vi "Set Bias Voltage.vi"(8 "error in (no error)":errorcluster, 9 "Channel":i32, 10 "Bias Voltage (V)":dbl, 11 "Example in":refnum<class "Instrument.Template.lvclass">) -> (0 "error out":errorcluster, 3 "Example out":refnum<class "Instrument.Template.lvclass">)   [LabVIEW 2019, in "Instrument.Template.lvclass"]
uses:
  Instrument.Template/Instrument.Template.lvclass
  Typedefs/Instrument.Template.Commands--Enum.ctl
  67792bfe-8e2c-4879-abc2-cb448bcec168.vi
  67792bfe-8e2c-4879-abc2-cb448bcec168.vi/c75e12d4-2661-49a5-9afc-dbffdb694870.vi
  67792bfe-8e2c-4879-abc2-cb448bcec168.vi/2a0bf3c4-890a-488b-bba9-7d0e50155bd9.vi
  67792bfe-8e2c-4879-abc2-cb448bcec168.vi/2a0bf3c4-890a-488b-bba9-7d0e50155bd9.vi/a640b9e0-2bb1-42d0-9491-26b19c1d8e7b.vi
  67792bfe-8e2c-4879-abc2-cb448bcec168.vi/2a0bf3c4-890a-488b-bba9-7d0e50155bd9.vi/8610e4ee-7e05-4c89-86eb-49a2000bc7ea.vi
  SMOs/RemoteControl/API/Remote Client.vi
  <vilib>/JDP Science/JSONtext/JSON text to Variant.vi
  <vilib>/JDP Science/JSONtext/LVClass Serializer/JSONtext LVClass Serializer.lvclass
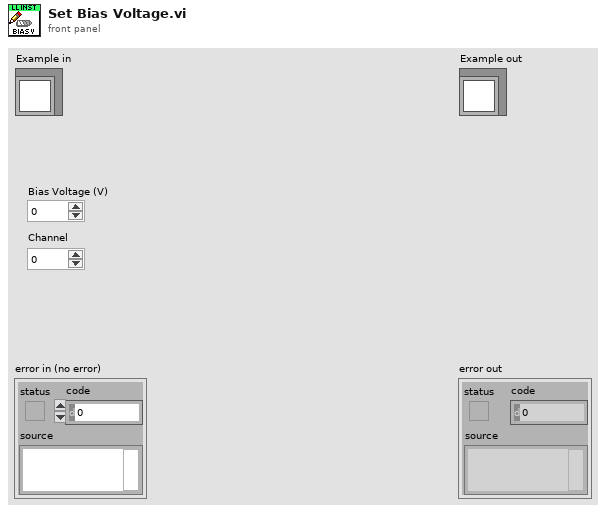
[diagram p1: front panel]
types:
  T1 = typedef "Instrument.Template.lvclass/Instrument.Template.Commands--Enum.ctl" = enum16{"command0", "command1", "command2"}
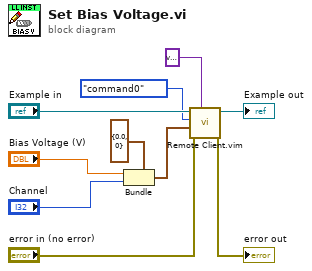
[diagram p0: block diagram]
diagram:
  n1 = Bundle(cluster=cluster{"Bias Voltage (V)":dbl, "Channel":i32} {"Bias Voltage (V)"=0.0, "Channel"=0} ("output cluster"), "Bias Voltage (V)"="Bias Voltage (V)", "Channel"="Channel") -> (w3:cluster{"Bias Voltage (V)":dbl, "Channel":i32})
  n2 = call "Remote Client.vim"("Data Out type"=variant, "error in (no error)"="error in (no error)", "params"=w3, "method"=Instrument.Template.Commands--Enum."command0" ("Commands"), "Instrument in"="Example in") -> ("error out"=→"error out":errorcluster, "Instrument out"=→"Example out":refnum<class "Instrument.Template.lvclass">)  [unwired: 3 in, 2 out]
